vi "Comments.Create Lockin Sampling Description.vi"(7 "error in (no error)":errorcluster, 10 "Control Experiment":refnum<class "Control Experiment.lvclass">) -> (0 "error out":errorcluster, 2 "Sampling Section":string, 3 "Control Experiment out":refnum<class "Control Experiment.lvclass">)   [LabVIEW 2016, in "Control Experiment.lvclass"]
uses:
  Control Experiment.lvclass
  Control Experiment.lvclass/Control Experiment.ctl
  <userlib>/LevyLab/Lockin-Multichannel/Instrument.Lockin/Instrument.Lockin.lvclass
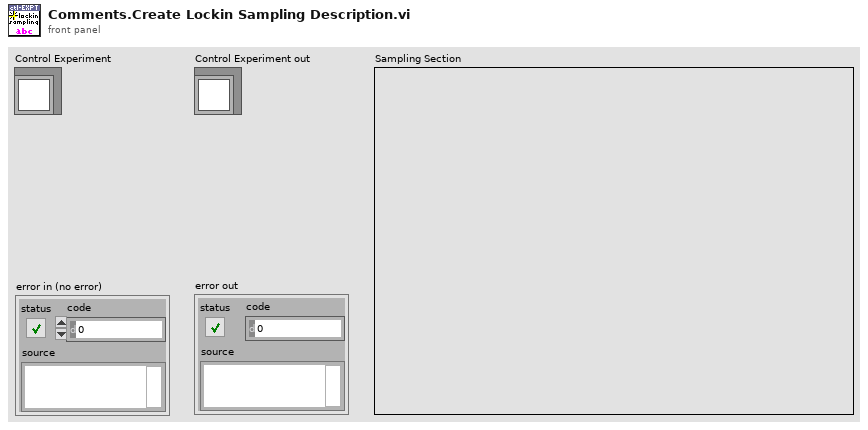
[diagram p1: front panel]
types:
  T1 = typedef "Instrument.Lockin.lvclass/Sampling.ctl" = cluster{"Fs":i32, "#s":i32}
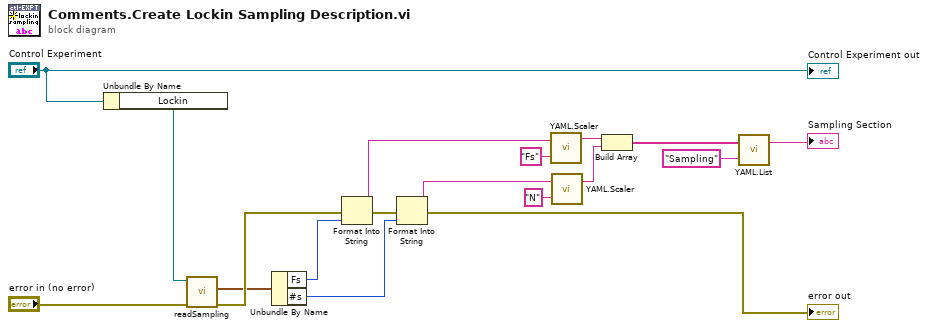
[diagram p0: block diagram]
diagram:
  n1 = Unbundle By Name("Control Experiment") -> ("Lockin"=w7:refnum<class "Instrument.Lockin.lvclass">)
  n2 = call <userlib>:"readSampling.vi"("error in (no error)"="error in (no error)", "Instrument.Lockin in"=w7) -> ("error out"=w6:errorcluster, "sampling"=w5:T1)  [unwired: 7 in, 1 out]
  n3 = Unbundle By Name(w5) -> ("Fs"=w17:i32, "#s"=w1:i32)
  n4 = Format Into String(error in=w6, w17) -> (resulting string=w10:string, error out=w18:errorcluster)  [unwired: 2 in]
  n5 = Format Into String(error in=w18, w1) -> (resulting string=w12:string, error out=→"error out":errorcluster)  [unwired: 2 in]
  n6 = call "YAML.Scaler.vi"("Key"="Fs", "Scaler"=w10) -> ("Output"=w4:string)  [unwired: 1 in]
  n7 = call "YAML.Scaler.vi"("Key"="N", "Scaler"=w12) -> ("Output"=w3:string)  [unwired: 1 in]
  n8 = Build Array(w4, w3) -> (w2:string[])
  n9 = call "YAML.List.vi"("Key"="Sampling" ("string"), "lines"=w2) -> ("Output"=→"Sampling Section":string)  [unwired: 1 in]
  "Control Experiment out" <- "Control Experiment"
